vi "Close Device.vi"(0 "niUsrpRio Session":T1={"FPGA Interface"=refnum, "RIO Interface Number"=0, "Data Clock Rate"=0, "FPGA Data Clock Rate"=0, "Global Settings Register Bus"=refnum, "Radio 0 Settings Register Bus"=refnum, "Radio 1 Settings Register Bus"=refnum, "Radio Settings Bus Semaphore"=refnum, "DB Queues"=[], "Characterization Data Valid?"=FALSE, "EEPROM Header"={"Checksum"=0, "Product Code"=0, "Hardware Current Version"=0, "Hardware Oldest Compatible Version"=0, "EEPROM Map Current Version"=0, "EEPROM Map Oldest Compatible Version"=0, "User Password"="", "Pointer to Factory Header"=0, "Pointer to User Header"=0, "Recommended Interval"=0, "Number of Reserved Bytes"=9, "Number of Daughterboards"=0, "Daughterboard IDs"=[], "Daughterboard Serial Numbers"=[]}, "Device Data Header"={"Checksum"=0, "Number of Channels"=0, "Number of Gain Settings"=[], "Pointer to Characterization Data"=[], "Number of Reserved Bytes"=27, "Number of Frequencies"=[]}, "EEPROM Characterization Header"={"Checksum"=0, "Date"=timestamp(0 s since 1904-01-01), "Temperature"=0.0, "Misc. Info"="", "Pointer to Device Data Header"=0, "Number of Reserved Bytes"=28}, "Characterization Data"=[], "FPGA Current Version"=0, "FPGA Oldest Compatible Version"=0, "Fixed Logic Current Version"=0, "Fixed Logic Oldest Compatible Version"=0, "FPGA Radio Settings Bus Current Version"=0, "FPGA Radio Settings Bus Oldest Compatible Version"=0, "FPGA Board Config Current Version"=0, "FPGA Board Config Oldest Compatible Version"=0, "Daughterboard Clock Rate"=0, "daughterboard configuration session handles"=[]} {"Daughterboard Clock Rate" format="%#.3pHz"; "FPGA Data Clock Rate" format="%#.3pHz"; "Data Clock Rate" format="%#.3pHz"; "Characterization Data"."Frequencies [Hz]" format="%#_6p"; "EEPROM Characterization Header"."Pointer to Device Data Header" format="%x"; "EEPROM Characterization Header"."Checksum" format="%x"; "Device Data Header"."Pointer to Characterization Data" format="%x"; "Device Data Header"."Checksum" format="%x"; "EEPROM Header"."Pointer to User Header" format="%x"; "EEPROM Header"."Pointer to Factory Header" format="%x"; "EEPROM Header"."Product Code" format="%x"; "EEPROM Header"."Checksum" format="%x"}, 11 "error in":errorcluster) -> (15 "error out":errorcluster)   [LabVIEW 2020]
doc: "Closes the niUsrpRio session to the device."
uses:
  <instrlib>/niUsrpRio/Config/v1/Host/Public/niUsrpRio Session.ctl
  <instrlib>/_niInstr/Register Bus/v0/Host/Public/Register Bus Session.ctl
  <instrlib>/_niInstr/Register Bus/v0/Host/Private/Session Data.ctl
  <instrlib>/niUsrpRio/Config/v1/Host/Private/DB Queue Reference.ctl
  <instrlib>/niUsrpRio/Config/v1/Host/Private/Daughterboard Data.ctl
  <instrlib>/niUsrpRio/Config/v1/Host/Private/ATR state data.ctl
  <instrlib>/niUsrpRio/Config/v1/Host/Private/Antenna Configuration.ctl
  <instrlib>/niUsrpRio/Config/v1/Host/Private/CPLD Power Mode.ctl
  <instrlib>/niUsrpRio/Config/v1/Host/Public/EEPROM Header.ctl
  <instrlib>/niUsrpRio/Config/v1/Host/Public/EEPROM Device Data Header.ctl
  <instrlib>/niUsrpRio/Config/v1/Host/Public/EEPROM Characterization Header.ctl
  <instrlib>/niUsrpRio/Config/v1/Host/Public/Characterization Data.ctl
  <instrlib>/niUsrpRio/Config/v1/Host/Public/IQ Imbalance.ctl
  <instrlib>/niUsrpRio/Config/v1/Host/Public/What to Query for.ctl
  <instrlib>/niUsrpRio/Config/v1/Host/Private/ATR Register Addresses.ctl
  <instrlib>/niUsrpRio/Instruction Synchronizer/v1/Host/Public/Reset Broadcast.vi
  <vilib>/FPGAPlugInAG/Dynamic/niLvFpga_Close_Dynamic.vi
  <vilib>/rvi/interface/nirviCloseFPGA/nirviCloseFPGA.xnode
  <instrlib>/niUsrpRio/Config/v1/Host/niUsrpRio Config v1 Host.lvlib
  <instrlib>/niUsrpRio/Instruction Synchronizer/v1/Host/niUsrpRio Instruction Synchronizer v1 Host.lvlib
  <instrlib>/_niInstr/Register Bus/v0/Host/niInstr Register Bus v0 Host.lvlib
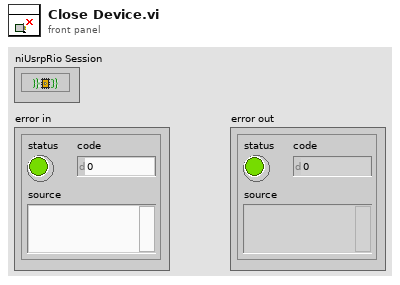
[diagram p1: front panel]
types:
  T1 = typedef "niUsrpRio Config v1 Host.lvlib/niUsrpRio Session.ctl" = cluster{"FPGA Interface":refnum<k20>, "RIO Interface Number":u32, "Data Clock Rate":u32, "FPGA Data Clock Rate":u32, "Global Settings Register Bus":T2, "Radio 0 Settings Register Bus":T2, "Radio 1 Settings Register Bus":T2, "Radio Settings Bus Semaphore":T3, "DB Queues":T4[], "Characterization Data Valid?":bool, "EEPROM Header":T5, "Device Data Header":T6, "EEPROM Characterization Header":T7, "Characterization Data":T8[], "FPGA Current Version":u32, "FPGA Oldest Compatible Version":u32, "Fixed Logic Current Version":u32, "Fixed Logic Oldest Compatible Version":u32, "FPGA Radio Settings Bus Current Version":u32, "FPGA Radio Settings Bus Oldest Compatible Version":u32, "FPGA Board Config Current Version":u32, "FPGA Board Config Oldest Compatible Version":u32, "Daughterboard Clock Rate":u32, "daughterboard configuration session handles":u64[]}
  T2 = typedef "niInstr Register Bus v0 Host.lvlib/Register Bus Session.ctl" = refnum<queue>
  T3 = typedef "Semaphore RefNum" = refnum<k1>
  T4 = typedef "niUsrpRio Config v1 Host.lvlib/DB Queue Reference.ctl" = refnum<queue>
  T5 = typedef "niUsrpRio Config v1 Host.lvlib/EEPROM Header.ctl" = cluster{"Checksum":u32, "Product Code":u16, "Hardware Current Version":u16, "Hardware Oldest Compatible Version":u16, "EEPROM Map Current Version":u16, "EEPROM Map Oldest Compatible Version":u16, "User Password":string, "Pointer to Factory Header":u32, "Pointer to User Header":u32, "Recommended Interval":u16, "Number of Reserved Bytes":i32, "Number of Daughterboards":u8, "Daughterboard IDs":u16[], "Daughterboard Serial Numbers":string[]}
  T6 = typedef "niUsrpRio Config v1 Host.lvlib/EEPROM Device Data Header.ctl" = cluster{"Checksum":u32, "Number of Channels":u8, "Number of Gain Settings":u16[], "Pointer to Characterization Data":u32[], "Number of Reserved Bytes":i32, "Number of Frequencies":u16[]}
  T7 = typedef "niUsrpRio Config v1 Host.lvlib/EEPROM Characterization Header.ctl" = cluster{"Checksum":u32, "Date":timestamp, "Temperature":sgl, "Misc. Info":string, "Pointer to Device Data Header":u32, "Number of Reserved Bytes":i32}
  T8 = typedef "niUsrpRio Config v1 Host.lvlib/Characterization Data.ctl" = cluster{"Gains[dB]":dbl[], "Frequencies [Hz]":dbl[], "IQ Imbalance Table":T9[], "Measured Gains[dB]":dbl[][]}
  T9 = typedef "niUsrpRio Config v1 Host.lvlib/IQ Imbalance.ctl" = cluster{"Gain Imbalance [linear]":dbl, "Phase Imbalance [radians]":dbl, "Offset":cdb}
  T10 = typedef "niUsrpRio Config v1 Host.lvlib/What to Query for.ctl" = enum16{"Clock Chip Lock Status", "Clock Chip Ever Unlocked", "LO Lock Status", "GPS Lock Status", "GPS Ever Unlocked", "DRAM Ready Status", "DAC PLL Lock Status", "DAC Sync Lock Status", "Data Clock PLL Lock Status", "Data Clock PLL Ever Unlocked", "ADC Clock PLL Lock Status", "ADC Clock PLL Ever Unlocked", "ADC Data Valid Status", "ADC Data Ever Invalid"}
  T11 = typedef "niUsrpRio Config v1 Host.lvlib/DB Types.ctl" = enum16{"sbx", "cbx", "wbx", "unknown", "ubx", "twinrx"}
  T12 = typedef "niUsrpRio Config v1 Host.lvlib/ATR Register Addresses.ctl" = u32
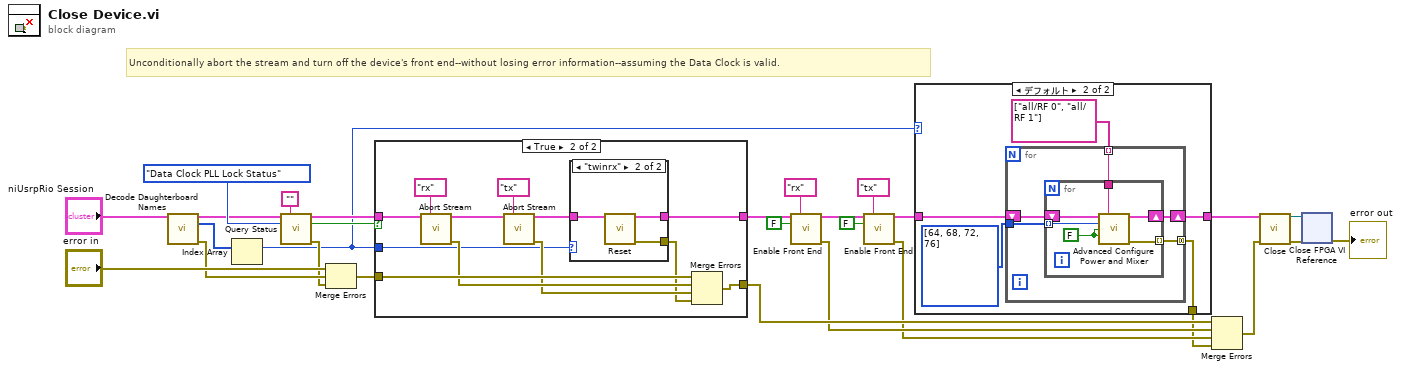
[diagram p0: block diagram]
diagram:
  # "Unconditionally abort the stream and turn off the device's front end--without losing error information--assuming the Data Clock is valid."
  n1 = call <instrlib>:"Decode Daughterboard Names.vi"("niUsrpRio Session"="niUsrpRio Session") -> ("niUsrpRio Session (out)"=w5:T1, "daughterboard names"=w4:T11[], "error out"=w3:errorcluster)  [unwired: 11 in, 1 out]
  n2 = Index Array(array=w4) -> (element=w1:T11)  [unwired: 1 in]
  n3 = call <instrlib>:"Query Status.vi"("niUsrpRio Session"=w5, "scope"="", "What to Query for"=What_to_Query_for."Data Clock PLL Lock Status") -> ("niUsrpRio Session (out)"=w17:T1, "Status"=w16:bool, "error out"=w2:errorcluster)  [unwired: 10 in]
  n4 = Merge Errors("error in", w3, w2) -> (w9:errorcluster)
  n5 = case shown="TRUE" w16 {
    tunnel: [w30 w34] -> w23
    tunnel: w17 -> [w30 w38]
    tunnel: w9 -> [w29 w42]
    tunnel: [w29 w37] -> w14
    tunnel: w1 -> [_ w32]
    frame False {
    }
    frame True {
      n6 = call "Abort Stream.vi"("niUsrpRio Session"=w38, "scope"="rx") -> ("niUsrpRio Session (out)"=w41:T1, "error out"=w36:errorcluster)  [unwired: 12 in]
      n7 = call "Abort Stream.vi"("niUsrpRio Session"=w41, "scope"="tx") -> ("niUsrpRio Session (out)"=w40:T1, "error out"=w35:errorcluster)  [unwired: 12 in]
      n8 = case shown="\"twinrx\"" w32 {
        tunnel: w40 -> [w43 w46]
        tunnel: [w43 w45] -> w34
        tunnel: [_ w44] -> w31
        frame Default {
        }
        frame "twinrx" {
          n9 = call-poly <instrlib>:"Reset.vi"("niUsrpRio Session"=w46) -> ("niUsrpRio Session (out)"=w45:T1, "error out"=w44:errorcluster)  [unwired: 13 in]
        }
      }
      n10 = Merge Errors(w42, w36, w35, w31) -> (w37:errorcluster)
    }
  }
  n11 = call <instrlib>:"Enable Front End.vi"("niUsrpRio Session"=w23, "scope"="rx", "enable"=FALSE) -> ("niUsrpRio Session (out)"=w22:T1, "error out"=w12:errorcluster)  [unwired: 11 in]
  n12 = call <instrlib>:"Enable Front End.vi"("niUsrpRio Session"=w22, "scope"="tx", "enable"=FALSE) -> ("niUsrpRio Session (out)"=w8:T1, "error out"=w11:errorcluster)  [unwired: 11 in]
  n13 = case shown="デフォルト" w1 {
    tunnel: w8 -> [w47 w50]
    tunnel: [w47 w49] -> w7
    tunnel: [_ w48] -> w6
    frame "twinrx" {
      # "TwinRx power and mixer cannot be controlled"
    }
    frame Default {
      w52 = T12[] [64, 68, 72, 76] items=["Idle"=64, "Rx Only"=68, "Tx Only"=72, "Full Duplex"=76] ("appended array")
      n14 = for {
        shift-right: [w56] -> w49
        shift-left: w50 -> [w57]
        tunnel: w52 -> [w55]
        tunnel: [w54] -> w48 mode=concatenating
        tunnel: string[] ["all/RF 0", "all/RF 1"] ("appended array") -> [w53] mode=indexing
        n15 = for {
          shift-right: [w62] -> w56
          shift-left: w57 -> [w63]
          tunnel: w55 -> [w61] mode=indexing
          tunnel: [w59] -> w54 mode=indexing
          tunnel: w53 -> [w58]
          w60 = FALSE ("power enable")
          n16 = call <instrlib>:"Advanced Configure Power and Mixer.vi"("niUsrpRio Session"=w63, "scope"=w58, "atr register"=w61, "power enable"=w60, "mixer enable"=w60) -> ("niUsrpRio Session (out)"=w62:T1, "error out"=w59:errorcluster)  [unwired: 9 in]
        }
      }
    }
  }
  n17 = Merge Errors(w14, w12, w11, w6) -> (w20:errorcluster)
  n18 = call <instrlib>:"Close.vi"("niUsrpRio Session"=w7, "error in"=w20) -> ("fpga ref (out)"=w28:refnum<k20>, "error out"=w19:errorcluster)  [unwired: 12 in]
  n19 = xnode "Close FPGA VI Reference"("FPGA VI Reference In"=w28, "error in"=w19) -> ("error out"=→"error out":errorcluster)
